vi "SPU_Set_Sampling_Parameter.vi"(0 "引用":refnum<k24>, 1 "startwave":dbl, 2 "stopwave":dbl, 3 "speed":dbl, 4 "triggerstep":dbl, 5 "错误输入（无错误）":errorcluster) -> (14 "引用输出":refnum<k24>, 19 "error IO":errorcluster)   [LabVIEW 2017]
uses:
  D:/test/PDLSTS/LV_PDL LvVer17.0/LV_PDL_x86/DLL/InstrumentDLL.dll
  DLL/InstrumentDLL.dll
  Share/MPM_PowerMonitorType.vi
  Share/Product_PCU.vi
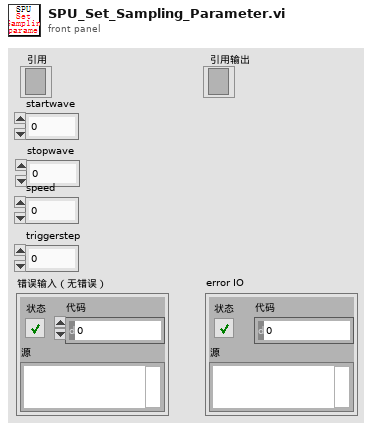
[diagram p1: front panel]
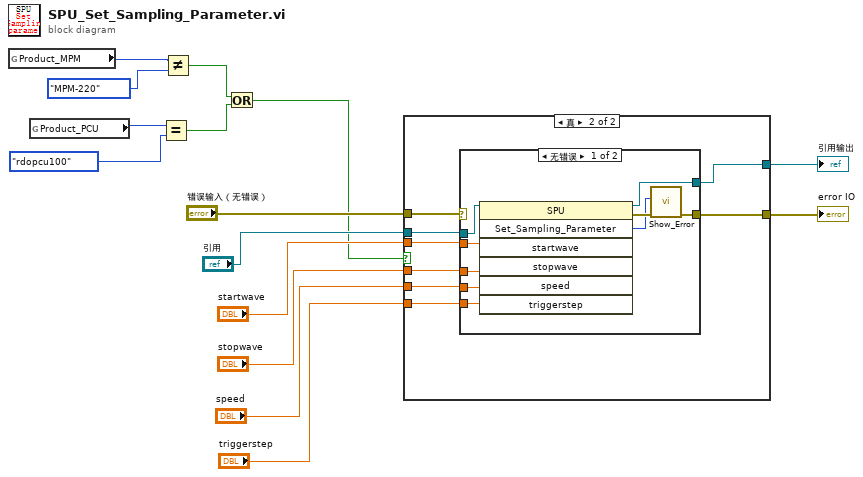
[diagram p0: block diagram]
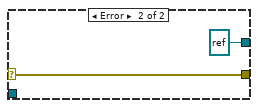
[diagram p3: hidden frame]
diagram:
  n1 = global read "MPM_PowerMonitorType.vi" "Product_MPM"() -> (w3:enum32{"MPM-210/210H", "MPM-220"})
  n2 = global read "Product_PCU.vi" "Product_PCU"() -> (w6:enum32{"rdopcu100", "rdopcu110"})
  n3 = Equal?(x=w6, y=enum32{"rdopcu100", "rdopcu110"}."rdopcu100" ("Product_PCU")) -> (x = y?=w7:bool)
  n4 = Not Equal?(x=w3, y=enum32{"MPM-210/210H", "MPM-220"}."MPM-220" ("Product_MPM")) -> (x != y?=w4:bool)
  n5 = Or(x=w4, y=w7) -> (x .or. y?=w1:bool)
  n6 = case shown="真" w1 {
    tunnel: "错误输入（无错误）" -> [w17 w25]
    tunnel: [w16 w24] -> w14
    tunnel: [w17 w23] -> w13
    tunnel: "引用" -> [w16 w22]
    tunnel: "startwave" -> [_ w21]
    tunnel: "stopwave" -> [_ w20]
    tunnel: "speed" -> [_ w19]
    tunnel: "triggerstep" -> [_ w18]
    frame False {
    }
    frame True {
      n7 = case shown="无错误" w25 {
        selector: w25 -> [_ w36]
        tunnel: [w32 w36] -> w23
        tunnel: [w31 refnum<k24> refnum ("new reference")] -> w24
        tunnel: w22 -> [w30 _]
        tunnel: w21 -> [w29 _]
        tunnel: w20 -> [w28 _]
        tunnel: w19 -> [w27 _]
        tunnel: w18 -> [w26 _]
        frame No Error {
          n8 = invoke class="SPU" method="Set_Sampling_Parameter"(reference=w30, "startwave"=w29, "stopwave"=w28, "speed"=w27, "triggerstep"=w26) -> (reference out=w31:refnum<k24>, error out=w34:errorcluster, "Set_Sampling_Parameter"=w33:i32)  [unwired: 2 in, 4 out]
          n9 = call "Show_Error.vi"("error in (no error)"=w34, "Error"=w33) -> ("error out"=w32:errorcluster)  [unwired: 9 in]
        }
        frame Error {
        }
      }
    }
  }
  "引用输出" <- w14
  "error IO" <- w13
